vi "Tank Do Stuffthings.vi"(8 "error in":errorcluster) -> (0 "error out":errorcluster, 1 "R Motor Power":dbl, 2 "Tank Mode":bool, 3 "L Motor Power":dbl)   [LabVIEW 2015]
uses:
  Support/Global Objects.vi
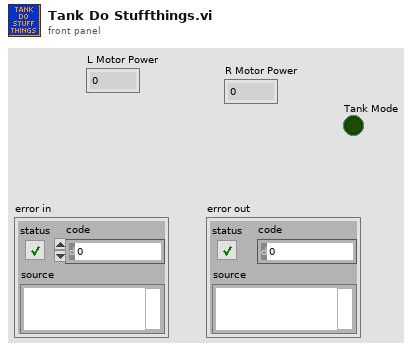
[diagram p1: front panel]
types:
  T1 = typedef "Teleop Commands.ctl" = cluster{"Throttle":dbl, "Turn":dbl, "Up Shift Commanded":bool, "Down Shift Commanded":bool, "Collect":bool, "Eject":bool, "Flywheel":bool, "Tank Mode":bool, "Left Motor Power":dbl, "Right Motor Power":dbl}
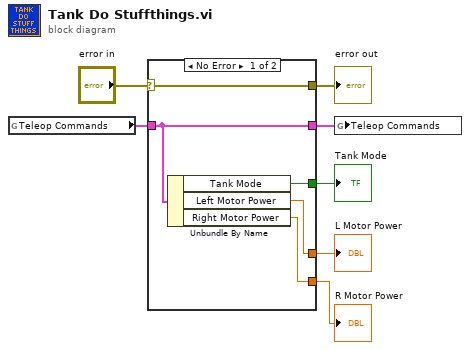
[diagram p0: block diagram]
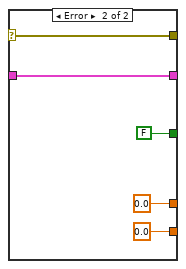
[diagram p2: hidden frame]
diagram:
  n1 = global read "Global Objects.vi" "Teleop Commands"() -> (w5:T1)
  n2 = case shown="No Error" "error in" {
    selector: "error in" -> [w12 w17]
    tunnel: [w12 w17] -> w6
    tunnel: [w11 w16] -> w4
    tunnel: w5 -> [w11 w16]
    tunnel: [w10 FALSE ("Collect")] -> w3
    tunnel: [w9 0.0 ("Left Motor Power")] -> w2
    tunnel: [w8 0.0 ("Right Motor Power")] -> w1
    frame No Error {
      n3 = Unbundle By Name(w11) -> ("Tank Mode"=w10:bool, "Left Motor Power"=w9:dbl, "Right Motor Power"=w8:dbl)
    }
    frame Error {
    }
  }
  "error out" <- w6
  "Tank Mode" <- w3
  "L Motor Power" <- w2
  "R Motor Power" <- w1
  n4 = global write "Global Objects.vi" "Teleop Commands"(w4) -> ()
